vi "WSVCAP SHL Host TL RFFE Write Cycle - Multiple DUTs - Common Data.vi"(0 "Data Out (Cycle Commands)":string[](array[string]), 5 "Post Command Delay":dbl[](array[numeric]) format="%#.0p s", 11 "error in":errorcluster, 13 "DUT Mask (All)":bool[](array[boolean])=[TRUE, TRUE, TRUE, TRUE, TRUE, TRUE, TRUE, TRUE, TRUE, TRUE, TRUE, TRUE, TRUE, TRUE, TRUE, TRUE, TRUE, TRUE, TRUE, TRUE, TRUE, TRUE, TRUE, TRUE, TRUE, TRUE, TRUE, TRUE, TRUE, TRUE, TRUE, TRUE, TRUE, TRUE, TRUE, TRUE], 14 "Log (T)":bool=TRUE) -> (15 "error out":errorcluster)   [LabVIEW 2012]
panel:
  out "Socket Mask":u64=1 format="%02x"
  out "RFFE Data Out [U8]":u8[][](array[numeric]) format="%02x"
  # "DUT 01"
  # "DUT 02"
  # "DUT 03"
  # "DUT 04"
  # "DUT 05"
  # "DUT 06"
  # "DUT 07"
  # "DUT 08"
  # "DUT 09"
  # "DUT 10"
  # "DUT 11"
  # "DUT 12"
  # "DUT 13"
  # "DUT 14"
  # "DUT 15"
  # "DUT 16"
  # "DUT 17"
  # "DUT 18"
  # "DUT 19"
  # "DUT 20"
  # "DUT 21"
  # "DUT 22"
  # "DUT 23"
  # "DUT 24"
  # "DUT 25"
  # "DUT 26"
  # "DUT 27"
  # "DUT 28"
  # "DUT 29"
  # "DUT 30"
  # "DUT 31"
  # "DUT 32"
  # "DUT 33"
  # "DUT 34"
  # "DUT 35"
  # "DUT 36"
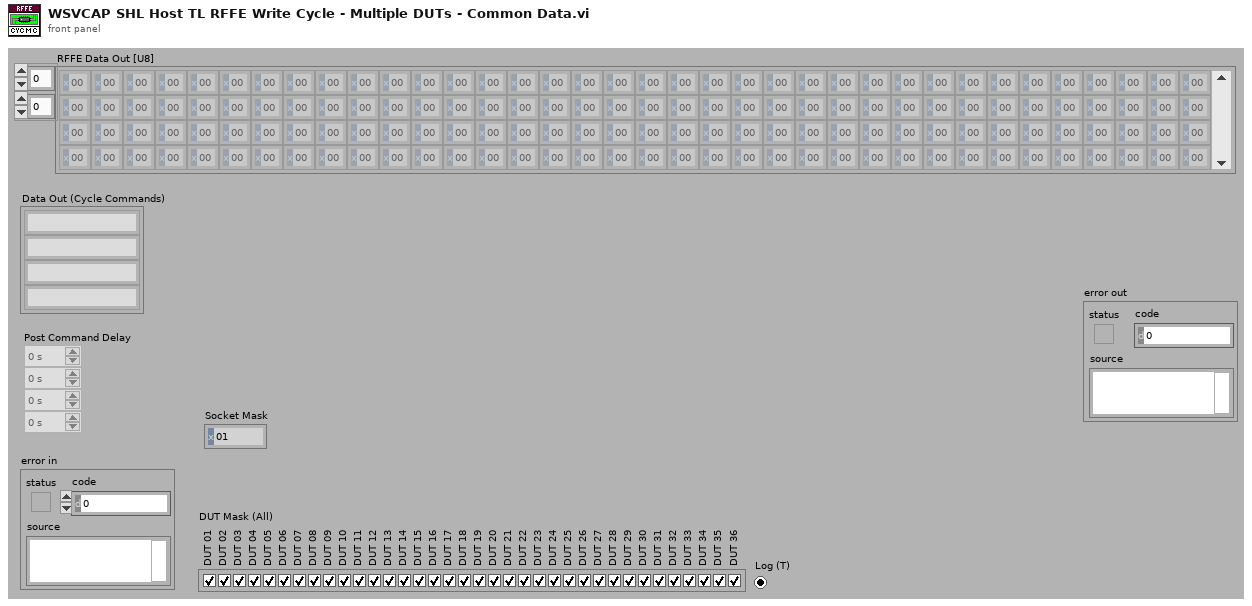
[diagram p1: front panel]
types:
  T1 = typedef "WSVCAP SHL Core System Cluster.ctl" = cluster{"Settings":T2, "FPGA Resource":tag, "Online":bool, "I2C Wait Ticks":u32, "SPI Wait Ticks":u32, "RFFE Wait Ticks":u32}
  T2 = typedef "WSVCAP SHL I2C Settings Cluster.ctl" = cluster{"FPGA Resource Name":string, "I2C Slave Address":u8, "I2C Clock Rate (Hz)":dbl, "SPI Clock Rate (Hz)":dbl, "RFFE Slave Address":u8, "RFFE Clock Rate (Hz)":dbl, "Simulate FPGA":bool, "C1 Cap DAC Default":u8, "C2 Cap DAC Default":u8, "C3 Cap DAC Default":u8}
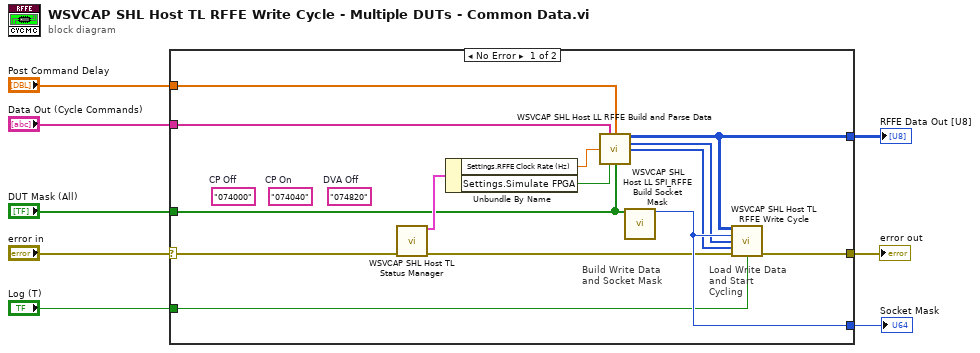
[diagram p0: block diagram]
diagram:
  n1 = case shown="No Error" "error in" {
    selector: "error in" -> [w9 _]
    tunnel: [w22 _] -> w8
    tunnel: [w21 _] -> w6
    tunnel: [w20 _] -> w5
    tunnel: "DUT Mask (All)" -> [w11 _]
    tunnel: "Post Command Delay" -> [w19 _]
    tunnel: "Data Out (Cycle Commands)" -> [w18 _]
    tunnel: "Log (T)" -> [w10 _]
    frame No Error {
      (unwired) "074820"  # DVA Off
      (unwired) "074040"  # CP On
      (unwired) "074000"  # CP Off
      # "Load Write Data and Start Cycling"
      # "Build Write Data and Socket Mask"
      n2 = call "WSVCAP SHL Host TL Status Manager.vi"("error in"=w9) -> ("System Out"=w17:T1, "error out"=w16:errorcluster)  [unwired: 13 in]
      n3 = Unbundle By Name(w17) -> ("Settings.RFFE Clock Rate (Hz)"=w12:dbl, "Settings.Simulate FPGA"=w15:bool)
      n4 = call "WSVCAP SHL Host LL RFFE Build and Parse Data.vi"("Data Out (Cycle Commands)"=w18, "Post Command Delay"=w19, "Clock Rate (Hz) (Cycle Only)"=w12, "Simulate FPGA (Cycle Only)"=w15, "DUT Mask (All)"=w11) -> ("RFFE Data Out [U8]"=w21:u8[][], "CMD Lengths (Bits)"=w14:u8[], "CMD Delays (Ticks)"=w13:u32[])  [unwired: 7 in, 1 out]
      n5 = call "WSVCAP SHL Host LL SPI_RFFE Build Socket Mask.vi"("DUT Mask"=w11) -> ("Socket Mask [U64]"=w20:u64)  [unwired: 14 in]
      n6 = call "WSVCAP SHL Host TL RFFE Write Cycle.vi"("RFFE Data Out"=w21, "Socket Mask"=w20, "Cycle CMD Lengths (bits)"=w14, "Cycle CMD Delay (ticks)"=w13, "error in"=w16, "Log (T)"=w10) -> ("error out"=w22:errorcluster)  [unwired: 9 in]
    }
    frame Error {
    }
  }
  "error out" <- w8
  "RFFE Data Out [U8]" <- w6
  "Socket Mask" <- w5
